vi "DashboardGet.vi"(10 "Joystick 2":T1, 11 "Joystick 1":T1) -> ()   [LabVIEW 2018]
uses:
  <vilib>/Rock Robotics/WPI/Joystick/WPI_JoystickDevRef.ctl
  <vilib>/Rock Robotics/WPI/Joystick/WPI_JoystickDeviceEnum.ctl
  RefNumsDriverStation.vi
  <vilib>/Rock Robotics/Network Tables/NT Read Boolean.vi
  Robot States.vi
  <vilib>/Rock Robotics/Network Tables/NT Read Number.vi
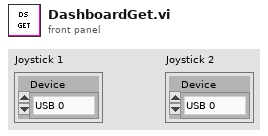
[diagram p1: front panel]
types:
  T1 = typedef "WPI_JoystickDevRef.ctl" = cluster{"Device":T2}
  T2 = typedef "WPI_JoystickDeviceEnum.ctl" = enum16{"USB 0", "USB 1", "USB 2", "USB 3", "USB 4", "USB 5"}
  T3 = cluster{"Boolean":bool, "Boolean":bool, "Boolean":bool, "Boolean":bool, "Boolean":bool, "Boolean":bool, "Boolean":bool}
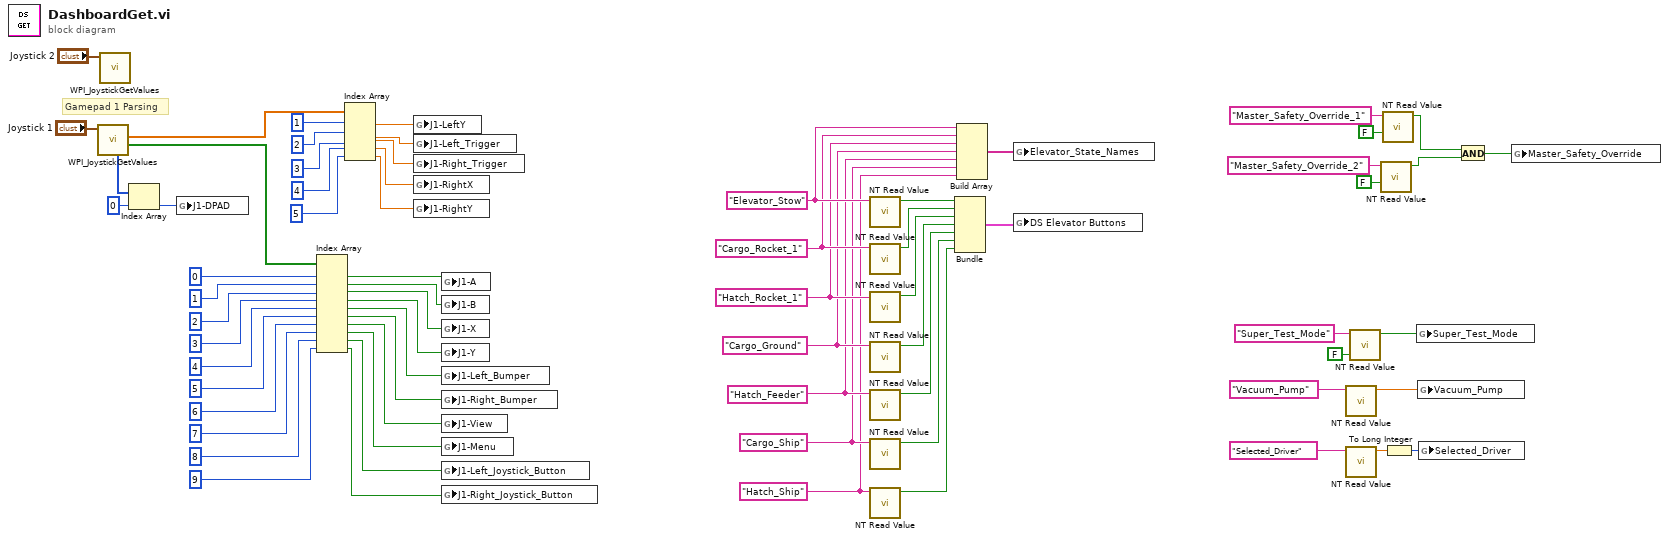
[diagram p0: block diagram]
diagram:
  w16 = "Hatch_Ship"
  w17 = "Cargo_Ship"
  w18 = "Hatch_Feeder"
  w19 = "Cargo_Ground"
  w20 = "Hatch_Rocket_1"
  w27 = "Cargo_Rocket_1"
  w30 = "Elevator_Stow"
  # "Gamepad 1 Parsing"
  n1 = call <vilib>:"WPI_JoystickGetValues.vi"("JoystickDevRef"="Joystick 1") -> ("Buttons"=w64:bool[], "Axes"=w65:dbl[], "POVs"=w68:i16[])  [unwired: 6 in, 2 out]
  n2 = call <vilib>:"WPI_JoystickGetValues.vi"("JoystickDevRef"="Joystick 2") -> ()  [unwired: 6 in, 5 out]
  n3 = Index Array(array=w68, index=0) -> (element=w66:i16)
  n4 = global write "RefNumsDriverStation.vi" "J1-DPAD"(w66) -> ()
  n5 = Index Array(array=w64, index #1=0 ("index"), index #2=1 ("index"), index #3=2 ("index"), index #4=3 ("index"), index #5=4 ("index"), index #6=5 ("index"), index #7=6 ("index"), index #8=7 ("index"), index #9=8 ("index"), index #10=9 ("index")) -> (element #1=w55:bool, element #2=w54:bool, element #3=w53:bool, element #4=w52:bool, element #5=w51:bool, element #6=w50:bool, element #7=w49:bool, element #8=w48:bool, element #9=w47:bool, element #10=w35:bool)
  n6 = Index Array(array=w65, index #1=1 ("index"), index #2=2 ("index"), index #3=3 ("index"), index #4=4 ("index"), index #5=5 ("index")) -> (element #1=w63:dbl, element #2=w56:dbl, element #3=w62:dbl, element #4=w61:dbl, element #5=w32:dbl)
  n7 = global write "RefNumsDriverStation.vi" "J1-LeftY"(w63) -> ()
  n8 = global write "RefNumsDriverStation.vi" "J1-Left_Trigger"(w56) -> ()
  n9 = global write "RefNumsDriverStation.vi" "J1-Right_Trigger"(w62) -> ()
  n10 = global write "RefNumsDriverStation.vi" "J1-RightX"(w61) -> ()
  n11 = global write "RefNumsDriverStation.vi" "J1-RightY"(w32) -> ()
  n12 = global write "RefNumsDriverStation.vi" "J1-A"(w55) -> ()
  n13 = global write "RefNumsDriverStation.vi" "J1-B"(w54) -> ()
  n14 = global write "RefNumsDriverStation.vi" "J1-X"(w53) -> ()
  n15 = global write "RefNumsDriverStation.vi" "J1-Y"(w52) -> ()
  n16 = global write "RefNumsDriverStation.vi" "J1-Left_Bumper"(w51) -> ()
  n17 = global write "RefNumsDriverStation.vi" "J1-Right_Bumper"(w50) -> ()
  n18 = global write "RefNumsDriverStation.vi" "J1-View"(w49) -> ()
  n19 = global write "RefNumsDriverStation.vi" "J1-Menu"(w48) -> ()
  n20 = global write "RefNumsDriverStation.vi" "J1-Left_Joystick_Button"(w47) -> ()
  n21 = global write "RefNumsDriverStation.vi" "J1-Right_Joystick_Button"(w35) -> ()
  n22 = call-poly <vilib>:"NT Read Value.vi"("Name"=w30) -> ("Boolean"=w28:bool)  [unwired: 9 in, 1 out]
  n23 = call-poly <vilib>:"NT Read Value.vi"("Name"=w27) -> ("Boolean"=w26:bool)  [unwired: 9 in, 1 out]
  n24 = call-poly <vilib>:"NT Read Value.vi"("Name"=w20) -> ("Boolean"=w25:bool)  [unwired: 9 in, 1 out]
  n25 = call-poly <vilib>:"NT Read Value.vi"("Name"=w19) -> ("Boolean"=w24:bool)  [unwired: 9 in, 1 out]
  n26 = call-poly <vilib>:"NT Read Value.vi"("Name"=w18) -> ("Boolean"=w23:bool)  [unwired: 9 in, 1 out]
  n27 = call-poly <vilib>:"NT Read Value.vi"("Name"=w17) -> ("Boolean"=w22:bool)  [unwired: 9 in, 1 out]
  n28 = call-poly <vilib>:"NT Read Value.vi"("Name"=w16) -> ("Boolean"=w21:bool)  [unwired: 9 in, 1 out]
  n29 = Bundle("Boolean"=w28, "Boolean"=w26, "Boolean"=w25, "Boolean"=w24, "Boolean"=w23, "Boolean"=w22, "Boolean"=w21) -> (w29:T3)  [unwired: 1 in]
  n30 = Build Array(w30, w27, w20, w19, w18, w17, w16) -> (w31:string[])
  n31 = global write "Robot States.vi" "Elevator_State_Names"(w31) -> ()
  n32 = global write "RefNumsDriverStation.vi" "DS Elevator Buttons"(w29) -> ()
  n33 = call-poly <vilib>:"NT Read Value.vi"("Name"="Vacuum_Pump") -> ("Numeric"=w11:dbl)  [unwired: 9 in, 1 out]
  n34 = call-poly <vilib>:"NT Read Value.vi"("Name"="Selected_Driver") -> ("Numeric"=w2:dbl)  [unwired: 9 in, 1 out]
  n35 = call-poly <vilib>:"NT Read Value.vi"("Default Value"=FALSE, "Name"="Super_Test_Mode") -> ("Boolean"=w13:bool)  [unwired: 8 in, 1 out]
  n36 = call-poly <vilib>:"NT Read Value.vi"("Default Value"=FALSE, "Name"="Master_Safety_Override_2") -> ("Boolean"=w5:bool)  [unwired: 8 in, 1 out]
  n37 = call-poly <vilib>:"NT Read Value.vi"("Default Value"=FALSE, "Name"="Master_Safety_Override_1") -> ("Boolean"=w6:bool)  [unwired: 8 in, 1 out]
  n38 = To Long Integer(number=w2) -> (32bit integer=w1:i32)
  n39 = global write "RefNumsDriverStation.vi" "Super_Test_Mode"(w13) -> ()
  n40 = global write "RefNumsDriverStation.vi" "Vacuum_Pump"(w11) -> ()
  n41 = global write "RefNumsDriverStation.vi" "Selected_Driver"(w1) -> ()
  n42 = And(x=w6, y=w5) -> (x .and. y?=w4:bool)
  n43 = global write "RefNumsDriverStation.vi" "Master_Safety_Override"(w4) -> ()
